vi "CopyFiles.vi"(8 "error in (no error)":errorcluster, 11 "Progress notifier":refnum<notifier>) -> (0 "error out":errorcluster, 3 "Progress notifier dup":refnum<notifier>)   [LabVIEW 2014, in "Installer.lvlib"]
uses:
  Installer.lvlib
  ProgressMessage.ctl
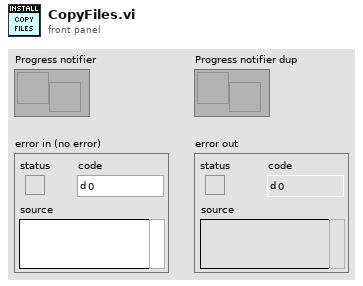
[diagram p1: front panel]
types:
  T1 = typedef "Installer.lvlib/ProgressMessage.ctl" = cluster{"Task":string, "Progress":i8}
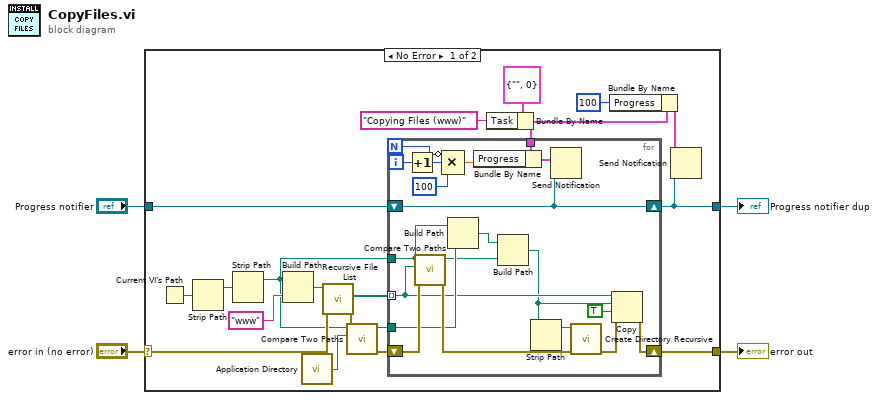
[diagram p0: block diagram]
diagram:
  n1 = case shown="No Error" "error in (no error)" {
    selector: "error in (no error)" -> [w21 w45]
    tunnel: [w20 w45] -> w3
    tunnel: "Progress notifier" -> [w11 w44]
    tunnel: [w8 w44] -> w1
    frame No Error {
      n2 = Current VI's Path() -> (path=w18:path)
      n3 = Strip Path(path=w18) -> (stripped path=w17:path)  [unwired: 1 out]
      n4 = Strip Path(path=w17) -> (stripped path=w13:path)  [unwired: 1 out]
      n5 = Build Path(base path=w13, name or relative path="www") -> (appended path=w14:path)
      n6 = call <vilib>:"Application Directory.vi"() -> ("Application Directory"=w12:path)
      n7 = call <vilib>:"Recursive File List.vi"("error in (no error)"=w21, "Folder Path"=w14) -> ("error out"=w23:errorcluster, "All Files in Dir"=w16:path[])  [unwired: 5 in, 3 out]
      n8 = call <vilib>:"Compare Two Paths.vi"("error in (no error)"=w23, "Path 2"=w12, "Path 1"=w13) -> ("error out"=w22:errorcluster, "Relative Path from 1 to 2"=w15:path)  [unwired: 5 in, 2 out]
      n9 = Bundle By Name(cluster=T1 {"Task"="", "Progress"=0} ("Progress Message"), "Task"="Copying Files (www)") -> (w7:T1)
      n10 = for {
        N -> [w31]
        tunnel: w16 -> [w35] mode=indexing
        tunnel: w15 -> [w38]
        tunnel: w13 -> [w39]
        shift-right: [w40] -> w20
        shift-left: w22 -> [w43]
        tunnel: w7 -> [w29]
        shift-right: [w26] -> w8
        shift-left: w11 -> [w26]
        i -> [w32]
        n11 = Increment(x=w32) -> (x+1=w30:i32)
        n12 = call <vilib>:"Compare Two Paths.vi"("error in (no error)"=w43, "Path 2"=w35, "Path 1"=w39) -> ("error out"=w42:errorcluster, "Relative Path from 1 to 2"=w36:path)  [unwired: 5 in, 2 out]
        n13 = Compound Arithmetic op=MULTIPLY(invert w31, w30, 100 ("value")) -> (w28:dbl)
        n14 = Build Path(base path=w39, name or relative path=w38) -> (appended path=w37:path)
        n15 = Bundle By Name(cluster=w29, "Progress"=w28) -> (w27:T1)
        n16 = Build Path(base path=w37, name or relative path=w36) -> (appended path=w34:path)
        n17 = Strip Path(path=w34) -> (stripped path=w33:path)  [unwired: 1 out]
        n18 = Send Notification(notification=w27, notifier=w26) -> ()  [unwired: 1 in, 2 out]
        n19 = call <vilib>:"Create Directory Recursive.vi"("error in (no error)"=w42, "directory"=w33) -> ("error out"=w41:errorcluster)  [unwired: 3 in, 2 out]
        n20 = Copy(8:w41, 9:TRUE ("overwrite (F)"), 10:w34, 11:w35) -> (0:w40:errorcluster)  [unwired: 1 in, 2 out]
      }
      n21 = Bundle By Name(cluster=w7, "Progress"=i8 100) -> (w5:T1)
      n22 = Send Notification(notification=w5, notifier=w8) -> ()  [unwired: 1 in, 2 out]
    }
    frame Error {
    }
  }
  "error out" <- w3
  "Progress notifier dup" <- w1
